vi "Local_Variable.vi"() -> ()   [LabVIEW 2022 SP3]
panel:
  out "Feihrheit":dbl(slide) scale=0.0..10.0
  in  "stop":bool
  out "Cilcius":dbl(slide) scale=0.0..10.0
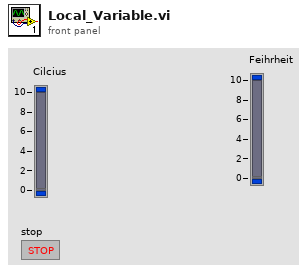
[diagram p1: front panel]
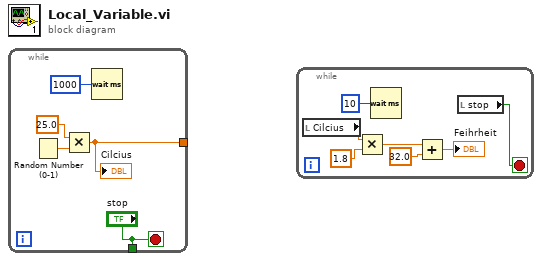
[diagram p0: block diagram]
diagram:
  n1 = while {
    tunnel: [w3] -> _
    tunnel: ["stop"] -> _
    stop <- "stop" stop-if-true
    n2 = Random Number (0-1)() -> (number: 0 to 1=w5:dbl)
    n3 = Multiply(x=25.0 ("y"), y=w5) -> (x*y=w3:dbl)
    "Cilcius" <- w3
    n4 = Wait (ms)(milliseconds to wait=u32 1000) -> ()  [unwired: 1 out]
  }
  n5 = while {
    stop <- w6 stop-if-true
    n6 = local read "Cilcius"() -> (w7:dbl)
    n7 = Multiply(x=w7, y=1.8) -> (x*y=w10:dbl)
    n8 = Wait (ms)(milliseconds to wait=u32 10) -> ()  [unwired: 1 out]
    n9 = Add(x=w10, y=32.0) -> (x+y=→"Feihrheit":dbl)
    n10 = local read "stop"() -> (w6:bool)
  }
